vi "GetModesOfOperation.vi"(8 "error in (no error)":errorcluster, 11 "Motor Base in":refnum<class "Motor Base.lvclass">) -> (0 "error out":errorcluster, 2 "Modes of operation":i8(ring)=8 items=["No mode change/no mode assigned"=0, "Profile position mode"=1, "Velocity mode"=2, "Profile velocity mode"=3, "Torque profile mode"=4, "Homing mode"=6, "Interpolated position mode"=7, "Cyclic synchronous position mode"=8, "Cyclic synchronous velocity mode"=9, "Cyclic synchronous torque mode"=10], 3 "Motor Base out":refnum<class "Motor Base.lvclass">)   [LabVIEW 2016, in "Motor Base.lvlib" / "Motor Base.lvclass"]
uses:
  Motor Base.lvclass
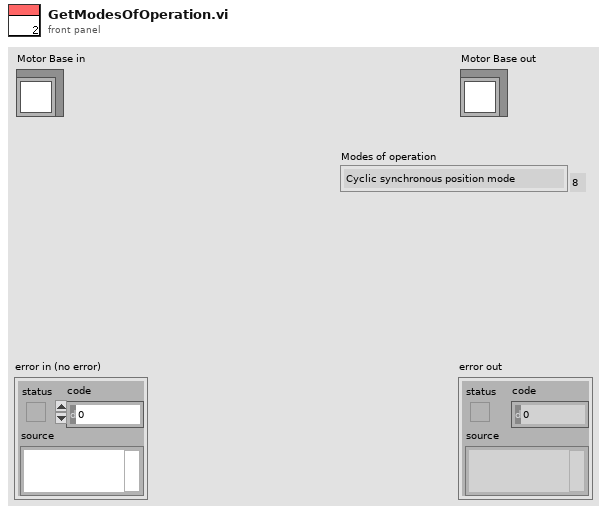
[diagram p1: front panel]
types:
  T1 = cluster{"Modes of operation":i8, "Feed(pulse)":u32, "Max motor speed(r/min)":u32, "Max torque(0.1%)":u16, "Min position limit(pulse)":i32, "Max position limit(pulse)":i32}
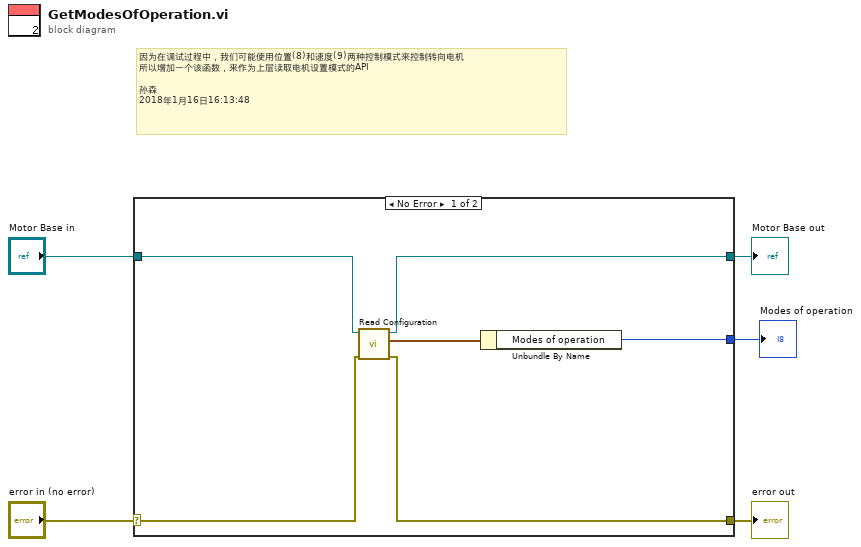
[diagram p0: block diagram]
diagram:
  # "因为在调试过程中，我们可能使用位置(8)和速度(9)两种控制模式来控制转向电机\n所以增加一个该函数，来作为上层读取电机设置模式的API\n\n孙森\n2018年1月16日16:13:48"
  n1 = case shown="No Error" "error in (no error)" {
    selector: "error in (no error)" -> [w9 w13]
    tunnel: [w8 w13] -> w4
    tunnel: [w10 w12] -> w2
    tunnel: "Motor Base in" -> [w11 w12]
    tunnel: [w6 _] -> w1
    frame No Error {
      n2 = call-dynamic "Read Configuration.vi"("error in (no error)"=w9, "Motor Base in"=w11) -> ("error out"=w8:errorcluster, "Configuration"=w7:T1, "Motor Base out"=w10:refnum<class "Motor Base.lvclass">)  [unwired: 7 in]
      n3 = Unbundle By Name(w7) -> ("Modes of operation"=w6:i8)
    }
    frame Error {
    }
  }
  "error out" <- w4
  "Motor Base out" <- w2
  "Modes of operation" <- w1
